vi "Format Bond Pad Points.vi"(6 "Bond Pad Groups":T2[](array[typedef]), 7 "Part Type":T1, 8 "error in":errorcluster, 9 "Slot":i32, 10 "Chuck":i32, 11 "Console Log in":refnum<class "Console Log.lvclass">) -> (0 "error out":errorcluster, 2 "Formatted Bond Pads":string[](array[string]), 3 "Console Log out":refnum<class "Console Log.lvclass">)   [LabVIEW 2011, in "Console Log.lvclass"]
uses:
  Console Log.lvclass
  Shared Components/Utils/Type Definitions/3d Line.ctl
  Shared Components/Vec3d Class/Vec3d Class.lvclass
  Shared Components/Config Manager Class/Type Definitions/Part Type.ctl
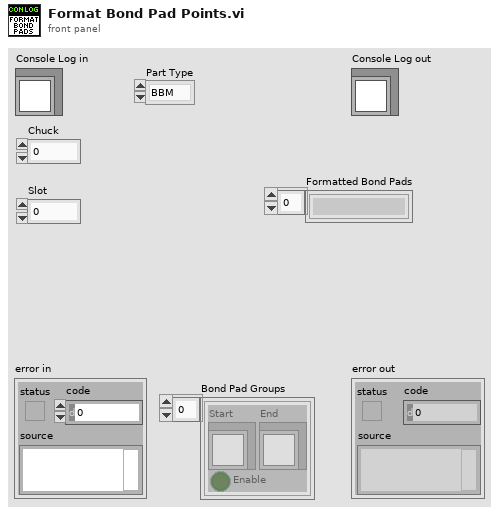
[diagram p1: front panel]
types:
  T1 = typedef "Part Type.ctl" = enum16{"BBM", "HDI", "GLUERESERVOIR", "STAMP", "WEIGHT"}
  T2 = typedef "3d Line.ctl" = cluster{"Start":refnum<class "Vec3d Class.lvclass">, "End":refnum<class "Vec3d Class.lvclass">, "Enable":bool}
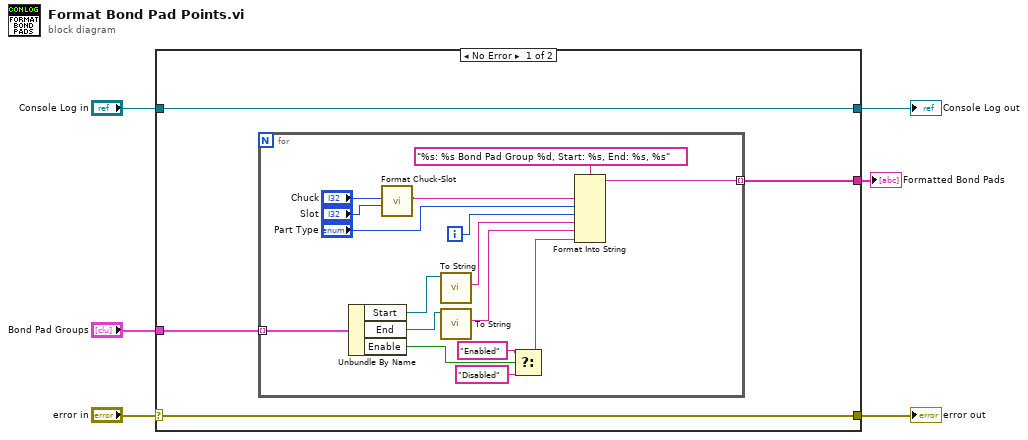
[diagram p0: block diagram]
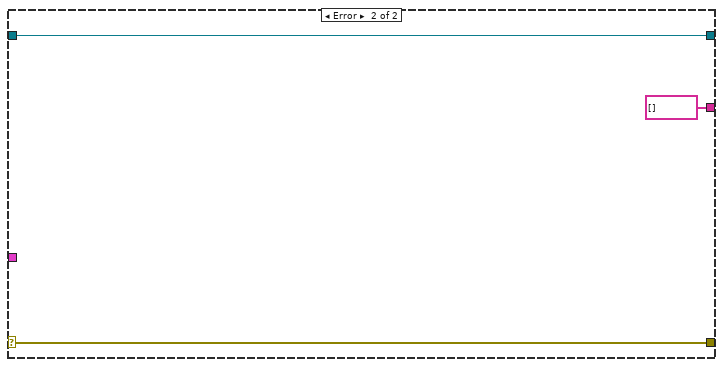
[diagram p2: hidden frame]
diagram:
  n1 = case shown="No Error" "error in" {
    selector: "error in" -> [w9 w29]
    tunnel: [w9 w29] -> w5
    tunnel: [w10 w28] -> w3
    tunnel: "Console Log in" -> [w10 w28]
    tunnel: "Bond Pad Groups" -> [w8 _]
    tunnel: [w7 string[] []] -> w1
    frame No Error {
      n2 = for {
        tunnel: w8 -> [w26] mode=indexing
        tunnel: [w14] -> w7 mode=indexing
        i -> [w19]
        n3 = Unbundle By Name(w26) -> ("Start"=w25:refnum<class "Vec3d Class.lvclass">, "End"=w24:refnum<class "Vec3d Class.lvclass">, "Enable"=w23:bool)
        n4 = call "Format Chuck-Slot.vi"("Slot"="Slot", "Chuck"="Chuck") -> ("Formatted Chuck/Slot"=w11:string)  [unwired: 7 in, 2 out]
        n5 = call "To String.vi"("Vec3d in"=w25) -> ("Vec3d String"=w18:string)  [unwired: 8 in, 2 out]
        n6 = call "To String.vi"("Vec3d in"=w24) -> ("Vec3d String"=w17:string)  [unwired: 8 in, 2 out]
        n7 = Select(t="Enabled", s=w23, f="Disabled") -> (s? t:f=w16:string)
        n8 = Format Into String(format string="%s: %s Bond Pad Group %d, Start: %s, End: %s, %s", w11, "Part Type", w19, w18, w17, w16) -> (resulting string=w14:string)  [unwired: 2 in, 1 out]
      }
    }
    frame Error {
    }
  }
  "error out" <- w5
  "Console Log out" <- w3
  "Formatted Bond Pads" <- w1
